vi "Wait.vi"(6 "time(0.1)":i32=100, 8 "error in (no error)":errorcluster, 9 "Wait?":bool=TRUE, 10 "Status":bool, 11 "FlowCtrl in":refnum<class "Station Action.lvclass">) -> (0 "error out":errorcluster, 1 "TimeOut":bool, 2 "StatusOut":bool, 3 "FlowCtrl out":refnum<class "Station Action.lvclass">)   [LabVIEW 2019, in "Station Action.lvclass"]
uses:
  Station Action.lvclass
  LLB/Commonly VI/Main Glb.vi
  LLB/Commonly VI.lvlib
  Ctrl/ModbusCmd.ctl
  FlowCtrl Class/BarcodeScan/Ctl/Board Scan IO.ctl
  Ctrl/S2 Station IO.ctl
  FlowCtrl Class/Laser Detect/Ctl/S11 Station IO.ctl
panel:
  in  "Boolean":bool=TRUE
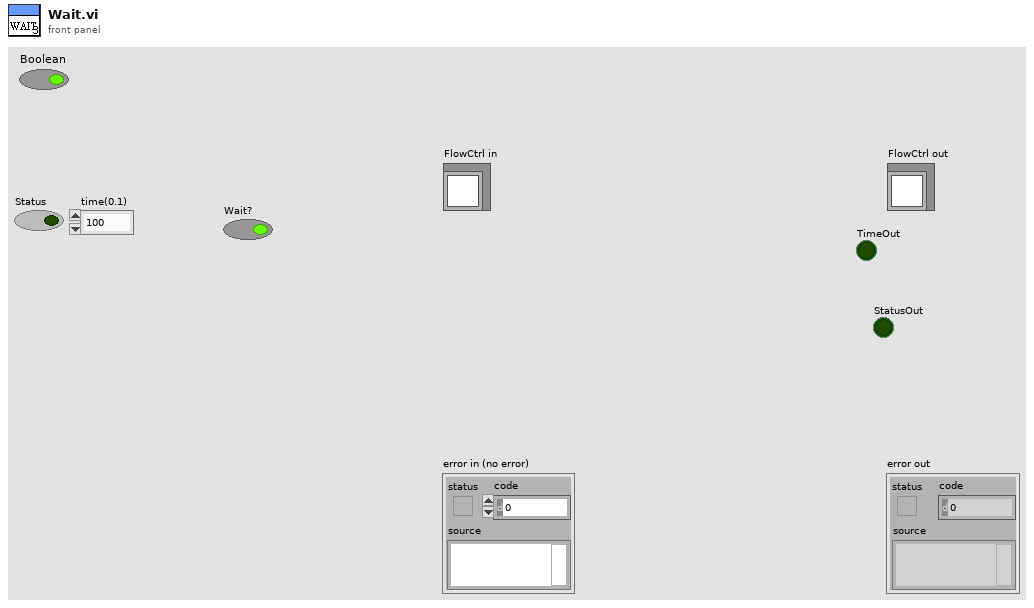
[diagram p1: front panel]
types:
  T1 = cluster{"starting address":u16, "number of inputs":u16, "Sat Coils":bool[], "Holding Registers":u16[]}
  T2 = typedef "ModbusCmd.ctl" = enum16{"Connect", "Disconnect", "Init", "Fetch Basic Objects", "Fetch Input Refisters", "Fetch Discrete Inputs", "Set Coils", "Set Holding Registers", "Write Single Holding", "Exit"}
  T3 = typedef "S2 Station IO.ctl" = enum16{"S2站PC動作中_20", "電流量測完成產品OK_21", "電流量測完成產品NG_22", "S2站Format 執行_23", "S2 Format OK_24", "S2 Format NG_25", "S2站燒入執行_26", "S2站燒入OK_27", "S2站燒入NG_28", "S2站動作完成_29", "S3 PC動作中_30", "S3 Format 此站執行_31", "S3 Format OK_32", "S3 Format NG_33", "S3 燒入程式 此站執行_34", "S3 燒入程式 OK_35", "S3 燒入程式 NG_36", "S3 備用_37", "S3 備用_38", "S3 動作完成_39", "S4 PC動作中_40", "S4 量測完成 產品正常_41", "S4 量測完成 產品NG_42", "S4 Format 此站執行_43", "S4 Format OK_44", "S4 Format NG_45", "S4 燒入 此站不執行_46", "S4 燒入程式 OK_47", "S4 燒入程式 NG_48", "S4 藍芽Scan OK_49", "S4 藍芽Scan NG_50", "S4 動作完成_51", "給PLC要量電流訊號", "給PLC要量電壓訊號"}
  T4 = typedef "Board Scan IO.ctl" = enum16{"S1 Barcode Scan", "回給PLC完成讀取訊號", "S1 載盤條碼比對NG", "S1PLC 條碼可讀取訊號", "S1備用_04", "S1備用_05", "S1備用_06", "S1備用_07", "S1備用_08", "S1 發送條碼完成"}
  T5 = typedef "S11 Station IO.ctl" = enum16{"S11雷射測量動作中", "S11雷射測點1完成", "S11雷射測點2完成", "S11雷測測量OK", "S11雷測測量NG", "S11雷測測量重測", "S11備用_6", "S11備用_7", "S11備用_8", "S11雷射測高完成"}
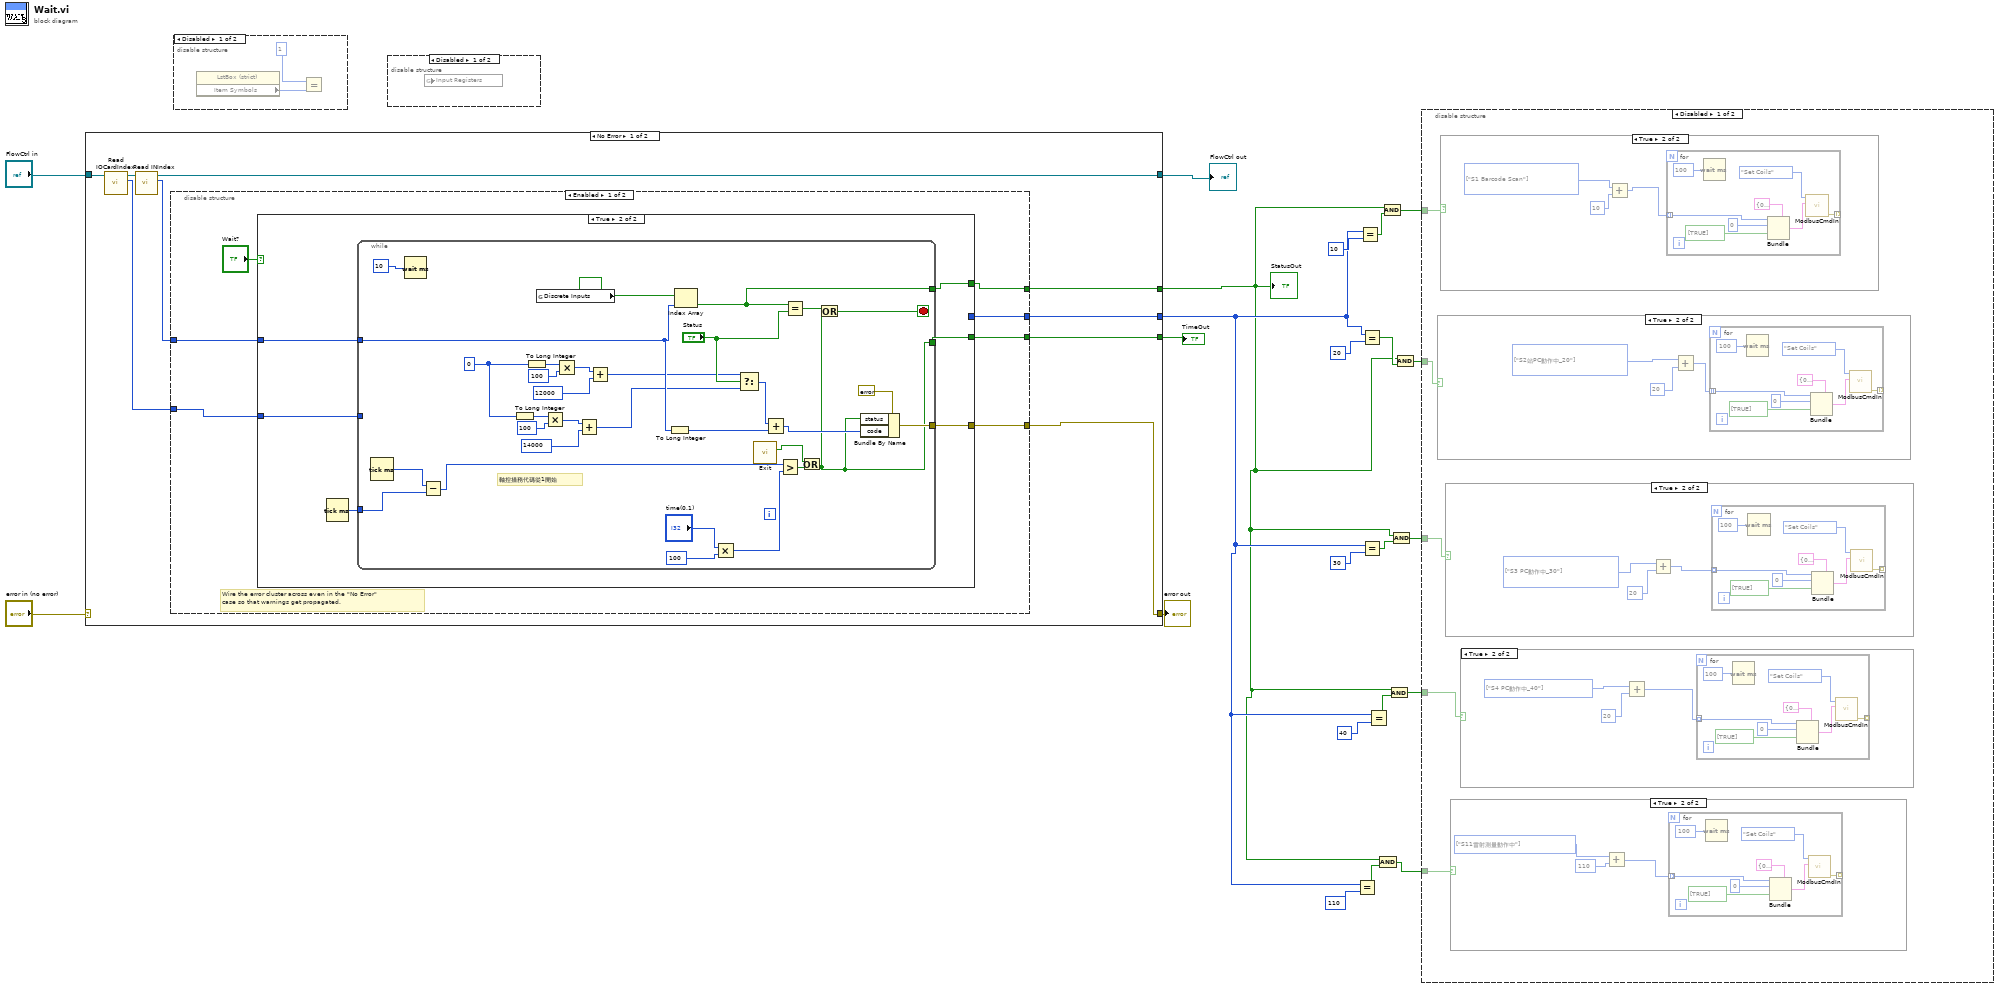
[diagram p0: block diagram]
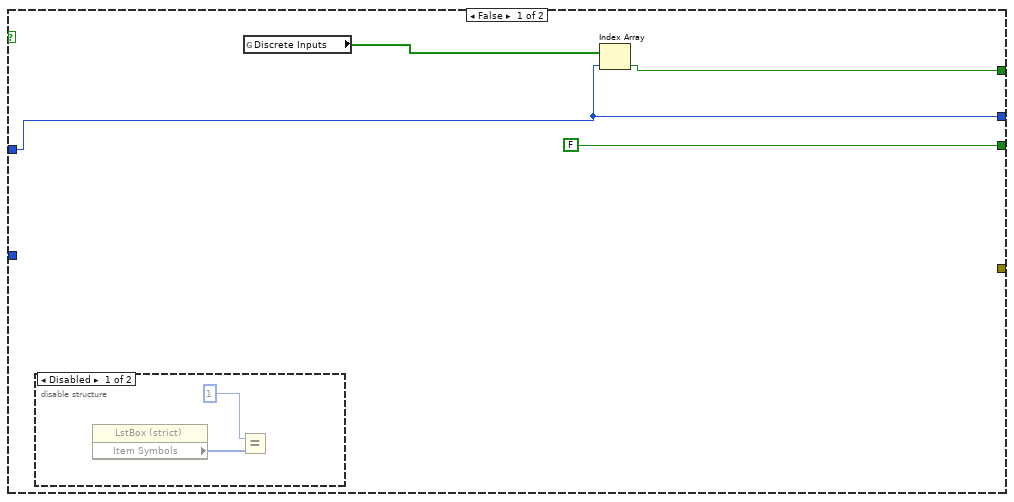
[diagram p10: hidden frame]
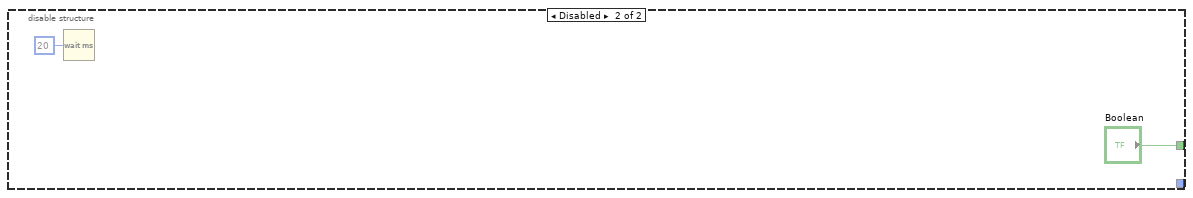
[diagram p12: hidden frame]
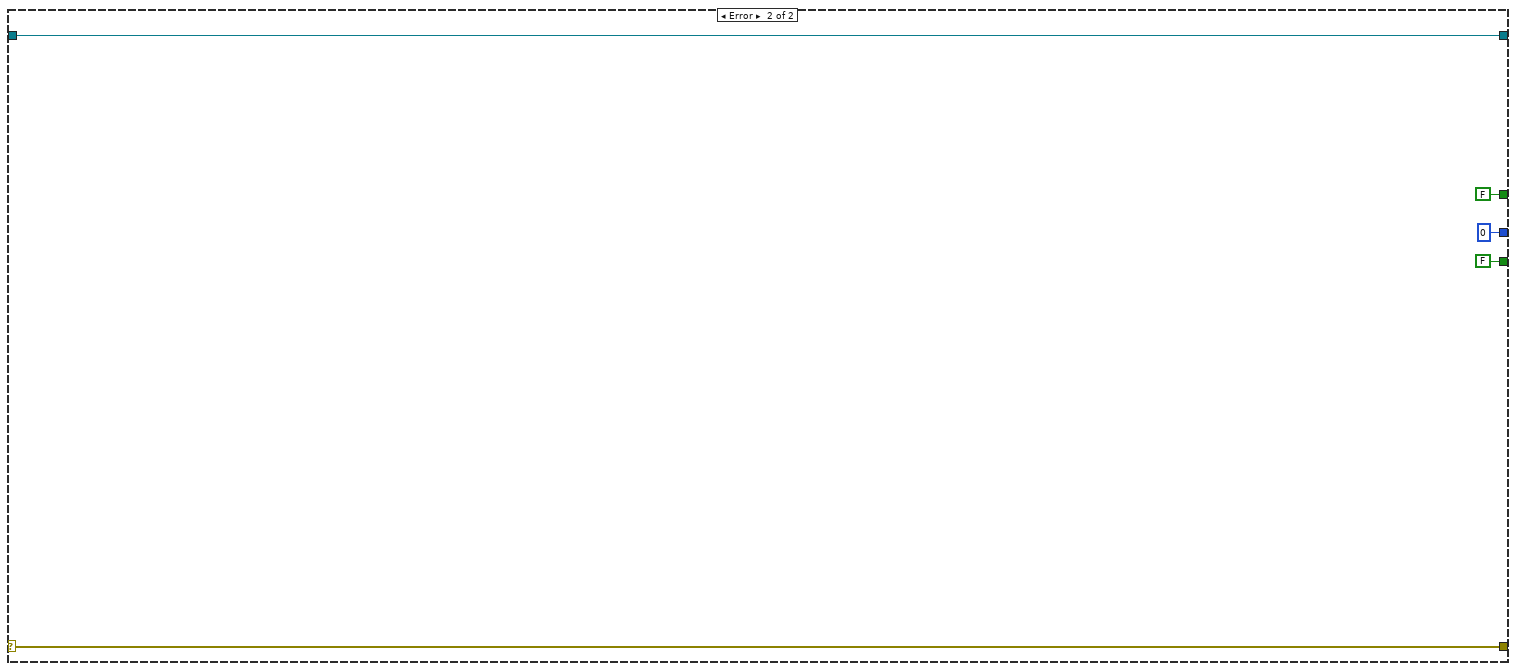
[diagram p13: hidden frame]
diagram:
  n1 = case shown="No Error" "error in (no error)" {
    selector: "error in (no error)" -> [_ w89]
    tunnel: [w26 w89] -> w21
    tunnel: [w28 w88] -> w19
    tunnel: "FlowCtrl in" -> [w31 w88]
    tunnel: [w25 FALSE] -> w18
    tunnel: [w24 FALSE] -> w3
    tunnel: [w23 0 ("INIndex")] -> w4
    frame No Error {
      n2 = call-dynamic "Read IOCardIndex.vi"("Station Action in"=w31) -> ("IOCardIndex"=w29:i32, "Station Action out"=w30:refnum<class "Station Action.lvclass">)  [unwired: 8 in, 1 out]
      n3 = call-dynamic "Read INIndex.vi"("Station Action in"=w30) -> ("INIndex"=w27:i32, "Station Action out"=w28:refnum<class "Station Action.lvclass">)  [unwired: 8 in, 1 out]
      n4 = disable-structure shown="Enabled" {
        disable-tunnel: w29 -> [w37 _]
        disable-tunnel: w27 -> [w36 _]
        disable-tunnel: [w35 _] -> w26
        disable-tunnel: [w34 _] -> w25
        disable-tunnel: [w33 "Boolean"] -> w24
        disable-tunnel: [w32 _] -> w23
        frame Enabled {
          # "Wire the error cluster across even in the \"No Error\"\ncase so that warnings get propagated."
          n5 = case shown="True" "Wait?" {
            tunnel: [FALSE w50] -> w34
            tunnel: [_ w49] -> w35
            tunnel: [w42 w48] -> w33
            tunnel: w36 -> [w39 w45]
            tunnel: w37 -> [_ w46]
            tunnel: [w39 _] -> w32
            frame False {
              n6 = disable-structure shown="Disabled" {
                frame Disabled {
                  n7 = property class="LstBox (strict)"() -> ("Item Symbols"=w43:i32[])  [unwired: 2 in, 2 out]
                  n8 = Equal?(x=1, y=w43) -> ()  [unwired: 1 out]
                }
                frame Enabled {
                }
              }
              n9 = global read "Main Glb.vi" "Discrete Inputs"() -> (w40:bool[])
              n10 = Index Array(array=w40, index=w39) -> (element=w42:bool)
            }
            frame True {
              n11 = Tick Count (ms)() -> (millisecond timer value=w47:u32)
              n12 = while {
                tunnel: [w73] -> w50
                tunnel: [w77] -> w49
                tunnel: [w55] -> w48
                tunnel: w45 -> [w72]
                tunnel: w47 -> [w57]
                tunnel: w46 -> [_]
                stop <- w81 stop-if-true
                w51 = 0 ("number")
                # "軸控措務代碼從1開始"
                n13 = Tick Count (ms)() -> (millisecond timer value=w58:u32)
                n14 = Wait (ms)(milliseconds to wait=u32 10) -> ()  [unwired: 1 out]
                n15 = Subtract(x=w58, y=w57) -> (x-y=w56:u32)
                n16 = To Long Integer(number=w51) -> (32bit integer=w63:i32)
                n17 = To Long Integer(number=w51) -> (32bit integer=w71:i32)
                n18 = global read "Main Glb.vi" "Discrete Inputs"() -> (w52:bool[])
                n19 = Multiply(x=w63, y=100) -> (x*y=w65:i32)
                n20 = Multiply(x=w71, y=100) -> (x*y=w69:i32)
                n21 = Add(x=w65, y=14000) -> (x+y=w62:i32)
                n22 = Add(x=w69, y=12000) -> (x+y=w67:i32)
                n23 = To Long Integer(number=w72) -> (32bit integer=w74:i32)
                n24 = Index Array(array=w52, index=w72) -> (element=w55:bool)
                n25 = Multiply(x="time(0.1)", y=u32 100 ("milliseconds to wait")) -> (x*y=w59:u32)
                n26 = Select(t=w67, s="Status", f=w62) -> (s? t:f=w75:i32)
                n27 = call "Exit.vi"() -> ("ExitOut"=w54:bool)  [unwired: 11 in]
                n28 = Add(x=w75, y=w74) -> (x+y=w78:i32)
                n29 = Greater?(x=w56, y=w59) -> (0:w79:bool)
                n30 = Equal?(x=w55, y="Status") -> (x = y?=w80:bool)
                n31 = Or(x=w54, y=w79) -> (x .or. y?=w73:bool)
                n32 = Compound Arithmetic op=OR(w80, w73) -> (w81:bool)
                n33 = Bundle By Name(cluster=errorcluster {"status"=FALSE, "code"=0, "source"=""} ("error Out"), "status"=w73, "code"=w78) -> (w77:errorcluster)
              }
            }
          }
        }
        frame Disabled {
          n34 = Wait (ms)(milliseconds to wait=u32 20) -> ()  [unwired: 1 out]
        }
      }
    }
    frame Error {
    }
  }
  "error out" <- w21
  "FlowCtrl out" <- w19
  "TimeOut" <- w18
  "StatusOut" <- w3
  n35 = disable-structure shown="Disabled" {
    frame Disabled {
      n36 = property class="LstBox (strict)"() -> ("Item Symbols"=w90:i32[])  [unwired: 2 in, 2 out]
      n37 = Equal?(x=1, y=w90) -> ()  [unwired: 1 out]
    }
    frame Enabled {
    }
  }
  n38 = disable-structure shown="Disabled" {
    frame Disabled {
      n39 = global read "Main Glb.vi" "Input Registers"() -> ()  [unwired: 1 in]
    }
    frame Enabled {
    }
  }
  n40 = Equal?(x=w4, y=110) -> (x = y?=w6:bool)
  n41 = Equal?(x=w4, y=10) -> (x = y?=w13:bool)
  n42 = Equal?(x=w4, y=20) -> (x = y?=w12:bool)
  n43 = Equal?(x=w4, y=30) -> (x = y?=w9:bool)
  n44 = Equal?(x=w4, y=40) -> (x = y?=w10:bool)
  n45 = And(x=w3, y=w6) -> (x .and. y?=w2:bool)
  n46 = And(x=w3, y=w13) -> (x .and. y?=w1:bool)
  n47 = And(x=w3, y=w10) -> (x .and. y?=w7:bool)
  n48 = And(x=w3, y=w9) -> (x .and. y?=w8:bool)
  n49 = And(x=w3, y=w12) -> (x .and. y?=w11:bool)
  n50 = disable-structure shown="Disabled" {
    disable-tunnel: w11 -> [w96 _]
    disable-tunnel: w8 -> [w95 _]
    disable-tunnel: w7 -> [w94 _]
    disable-tunnel: w2 -> [w93 _]
    disable-tunnel: w1 -> [w92 _]
    frame Disabled {
      n51 = case shown="True" w96 {
        frame False {
        }
        frame True {
          w131 = T3[] [enum."S2站PC動作中_20"] items=["S2站PC動作中_20", "電流量測完成產品OK_21", "電流量測完成產品NG_22", "S2站Format 執行_23", "S2 Format OK_24", "S2 Format NG_25", "S2站燒入執行_26", "S2站燒入OK_27", "S2站燒入NG_28", "S2站動作完成_29", "S3 PC動作中_30", "S3 Format 此站執行_31", "S3 Format OK_32", "S3 Format NG_33", "S3 燒入程式 此站執行_34", "S3 燒入程式 OK_35", "S3 燒入程式 NG_36", "S3 備用_37", "S3 備用_38", "S3 動作完成_39", "S4 PC動作中_40", "S4 量測完成 產品正常_41", "S4 量測完成 產品NG_42", "S4 Format 此站執行_43", "S4 Format OK_44", "S4 Format NG_45", "S4 燒入 此站不執行_46", "S4 燒入程式 OK_47", "S4 燒入程式 NG_48", "S4 藍芽Scan OK_49", "S4 藍芽Scan NG_50", "S4 動作完成_51", "給PLC要量電流訊號", "給PLC要量電壓訊號"]
          n52 = Add(x=w131, y=20) -> (x+y=w130:i32[])
          n53 = for {
            tunnel: [w134] -> _ mode=indexing
            tunnel: w130 -> [w133] mode=indexing
            n54 = Wait (ms)(milliseconds to wait=100) -> ()  [unwired: 1 out]
            n55 = Bundle(cluster=T1 {"starting address"=0, "number of inputs"=0, "Sat Coils"=[], "Holding Registers"=[]} ("data"), "starting address"=w133, "number of inputs"=u16 0, "Sat Coils"=bool[] [TRUE]) -> (w137:T1)  [unwired: 1 in]
            n56 = call "ModbusCmdIn.vi"("data"=w137, "Enum"=ModbusCmd."Set Coils") -> ("error out"=w134:errorcluster)  [unwired: 9 in]
          }
        }
      }
      n57 = case shown="True" w92 {
        frame False {
        }
        frame True {
          w142 = T4[] [enum."S1 Barcode Scan"] items=["S1 Barcode Scan", "回給PLC完成讀取訊號", "S1 載盤條碼比對NG", "S1PLC 條碼可讀取訊號", "S1備用_04", "S1備用_05", "S1備用_06", "S1備用_07", "S1備用_08", "S1 發送條碼完成"]
          n58 = Add(x=w142, y=10) -> (x+y=w143:i32[])
          n59 = for {
            tunnel: [w145] -> _ mode=indexing
            tunnel: w143 -> [w144] mode=indexing
            n60 = Wait (ms)(milliseconds to wait=100) -> ()  [unwired: 1 out]
            n61 = Bundle(cluster=T1 {"starting address"=0, "number of inputs"=0, "Sat Coils"=[], "Holding Registers"=[]} ("data"), "starting address"=w144, "number of inputs"=u16 0, "Sat Coils"=bool[] [TRUE]) -> (w148:T1)  [unwired: 1 in]
            n62 = call "ModbusCmdIn.vi"("data"=w148, "Enum"=ModbusCmd."Set Coils") -> ("error out"=w145:errorcluster)  [unwired: 9 in]
          }
        }
      }
      n63 = case shown="True" w95 {
        frame False {
        }
        frame True {
          w121 = T3[] [enum."S3 PC動作中_30"] items=["S2站PC動作中_20", "電流量測完成產品OK_21", "電流量測完成產品NG_22", "S2站Format 執行_23", "S2 Format OK_24", "S2 Format NG_25", "S2站燒入執行_26", "S2站燒入OK_27", "S2站燒入NG_28", "S2站動作完成_29", "S3 PC動作中_30", "S3 Format 此站執行_31", "S3 Format OK_32", "S3 Format NG_33", "S3 燒入程式 此站執行_34", "S3 燒入程式 OK_35", "S3 燒入程式 NG_36", "S3 備用_37", "S3 備用_38", "S3 動作完成_39", "S4 PC動作中_40", "S4 量測完成 產品正常_41", "S4 量測完成 產品NG_42", "S4 Format 此站執行_43", "S4 Format OK_44", "S4 Format NG_45", "S4 燒入 此站不執行_46", "S4 燒入程式 OK_47", "S4 燒入程式 NG_48", "S4 藍芽Scan OK_49", "S4 藍芽Scan NG_50", "S4 動作完成_51", "給PLC要量電流訊號", "給PLC要量電壓訊號"]
          n64 = Add(x=w121, y=20) -> (x+y=w119:i32[])
          n65 = for {
            tunnel: [w123] -> _ mode=indexing
            tunnel: w119 -> [w122] mode=indexing
            n66 = Wait (ms)(milliseconds to wait=100) -> ()  [unwired: 1 out]
            n67 = Bundle(cluster=T1 {"starting address"=0, "number of inputs"=0, "Sat Coils"=[], "Holding Registers"=[]} ("data"), "starting address"=w122, "number of inputs"=u16 0, "Sat Coils"=bool[] [TRUE]) -> (w126:T1)  [unwired: 1 in]
            n68 = call "ModbusCmdIn.vi"("data"=w126, "Enum"=ModbusCmd."Set Coils") -> ("error out"=w123:errorcluster)  [unwired: 9 in]
          }
        }
      }
      n69 = case shown="True" w93 {
        frame False {
        }
        frame True {
          w98 = T5[] [enum."S11雷射測量動作中"] items=["S11雷射測量動作中", "S11雷射測點1完成", "S11雷射測點2完成", "S11雷測測量OK", "S11雷測測量NG", "S11雷測測量重測", "S11備用_6", "S11備用_7", "S11備用_8", "S11雷射測高完成"]
          n70 = Add(x=w98, y=110) -> (x+y=w97:i32[])
          n71 = for {
            tunnel: [w101] -> _ mode=indexing
            tunnel: w97 -> [w100] mode=indexing
            n72 = Wait (ms)(milliseconds to wait=100) -> ()  [unwired: 1 out]
            n73 = Bundle(cluster=T1 {"starting address"=0, "number of inputs"=0, "Sat Coils"=[], "Holding Registers"=[]} ("data"), "starting address"=w100, "number of inputs"=u16 0, "Sat Coils"=bool[] [TRUE]) -> (w104:T1)  [unwired: 1 in]
            n74 = call "ModbusCmdIn.vi"("data"=w104, "Enum"=ModbusCmd."Set Coils") -> ("error out"=w101:errorcluster)  [unwired: 9 in]
          }
        }
      }
      n75 = case shown="True" w94 {
        frame False {
        }
        frame True {
          w109 = T3[] [enum."S4 PC動作中_40"] items=["S2站PC動作中_20", "電流量測完成產品OK_21", "電流量測完成產品NG_22", "S2站Format 執行_23", "S2 Format OK_24", "S2 Format NG_25", "S2站燒入執行_26", "S2站燒入OK_27", "S2站燒入NG_28", "S2站動作完成_29", "S3 PC動作中_30", "S3 Format 此站執行_31", "S3 Format OK_32", "S3 Format NG_33", "S3 燒入程式 此站執行_34", "S3 燒入程式 OK_35", "S3 燒入程式 NG_36", "S3 備用_37", "S3 備用_38", "S3 動作完成_39", "S4 PC動作中_40", "S4 量測完成 產品正常_41", "S4 量測完成 產品NG_42", "S4 Format 此站執行_43", "S4 Format OK_44", "S4 Format NG_45", "S4 燒入 此站不執行_46", "S4 燒入程式 OK_47", "S4 燒入程式 NG_48", "S4 藍芽Scan OK_49", "S4 藍芽Scan NG_50", "S4 動作完成_51", "給PLC要量電流訊號", "給PLC要量電壓訊號"]
          n76 = Add(x=w109, y=20) -> (x+y=w108:i32[])
          n77 = for {
            tunnel: [w112] -> _ mode=indexing
            tunnel: w108 -> [w111] mode=indexing
            n78 = Wait (ms)(milliseconds to wait=100) -> ()  [unwired: 1 out]
            n79 = Bundle(cluster=T1 {"starting address"=0, "number of inputs"=0, "Sat Coils"=[], "Holding Registers"=[]} ("data"), "starting address"=w111, "number of inputs"=u16 0, "Sat Coils"=bool[] [TRUE]) -> (w115:T1)  [unwired: 1 in]
            n80 = call "ModbusCmdIn.vi"("data"=w115, "Enum"=ModbusCmd."Set Coils") -> ("error out"=w112:errorcluster)  [unwired: 9 in]
          }
        }
      }
    }
    frame Enabled {
    }
  }
